vi "Event Logger.vi"(4 "Error IN":errorcluster, 7 "Main VI Base Path IN":path) -> (0 "Error OUT":errorcluster)   [LabVIEW 2018]
uses:
  <vilib>/Utility/file.llb/Write Delimited Spreadsheet (string).vi
  Globals/Global - Configuration Options.vi
panel:
  in  "Headers":string[](array[string])=["Date_Time", "Log Type", "Message"]
  out "Event Log Path":path
  # "INPUTS"
  # "OUTPUTS"
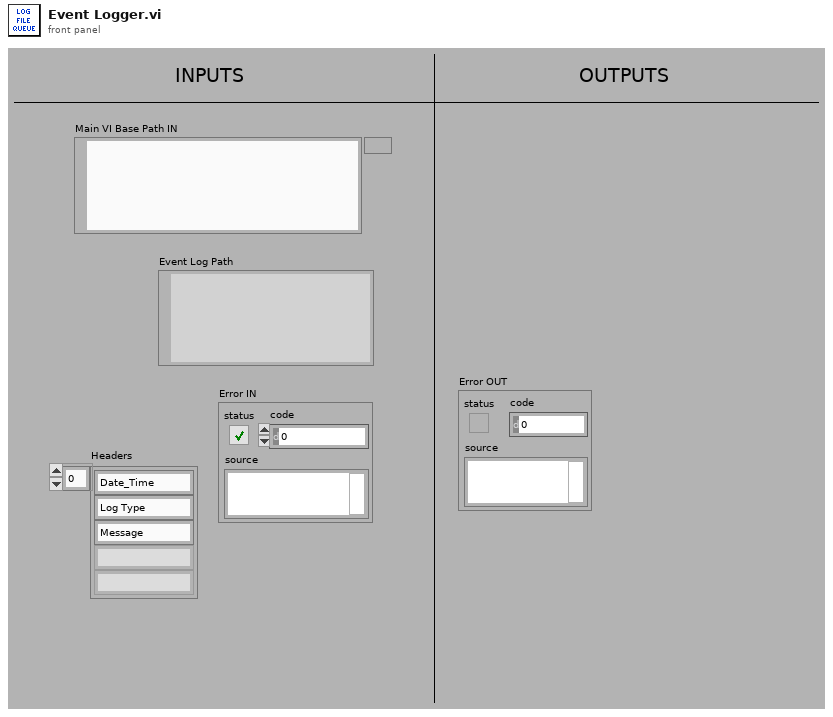
[diagram p1: front panel]
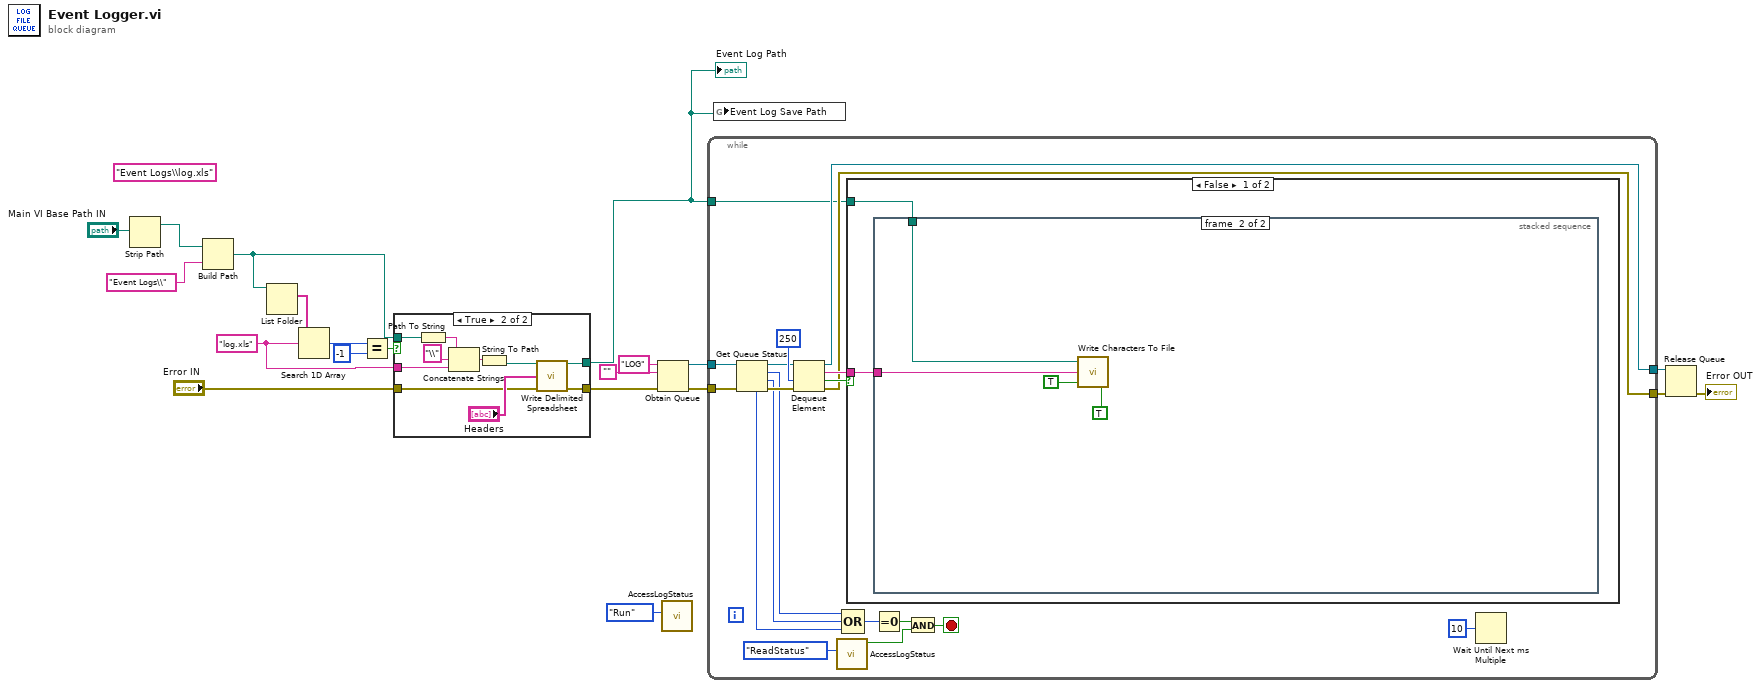
[diagram p0: block diagram]
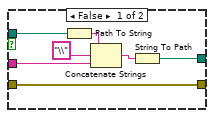
[diagram p2: hidden frame]
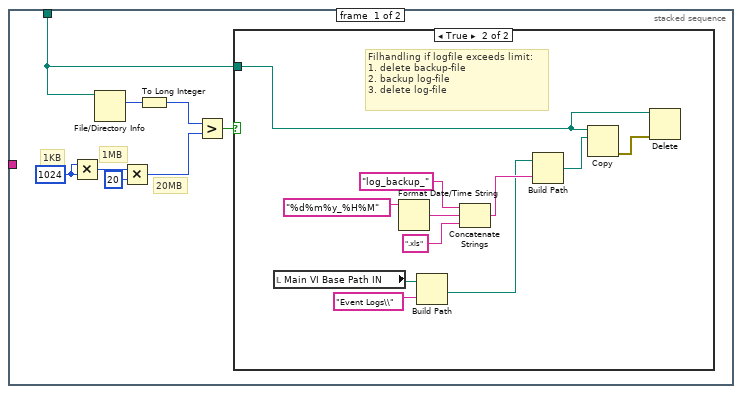
[diagram p3: hidden frame]
diagram:
  (unwired) "Event Logs\\log.xls" ("name or relative path")
  w8 = "log.xls" ("name or relative path")
  n1 = Strip Path(path="Main VI Base Path IN") -> (stripped path=w1:path)  [unwired: 1 out]
  n2 = Build Path(base path=w1, name or relative path="Event Logs\\") -> (appended path=w7:path)
  n3 = List Folder(path=w7) -> (filenames=w4:string[])  [unwired: 1 in, 5 out]
  n4 = Search 1D Array(1D array=w4, element=w8) -> (index of element=w11:i32)  [unwired: 1 out]
  n5 = Equal?(x=w11, y=-1) -> (x = y?=w9:bool)
  n6 = case shown="True" w9 {
    tunnel: w8 -> [w23 w37]
    tunnel: "Error IN" -> [w27 w28]
    tunnel: [w27 w31] -> w6
    tunnel: w7 -> [w21 w35]
    tunnel: [w22 w30] -> w3
    frame False {
      n7 = Path To String(path=w21) -> (string=w25:string)
      n8 = Concatenate Strings(w25, "\\", w23) -> (w26:string)
      n9 = String To Path(string=w26) -> (path=w22:path)
    }
    frame True {
      n10 = Path To String(path=w35) -> (string=w34:string)
      n11 = Concatenate Strings(w34, "\\", w37) -> (w36:string)
      n12 = String To Path(string=w36) -> (path=w29:path)
      n13 = call-poly <vilib>:"Write Delimited Spreadsheet.vi"("file path (dialog if empty)"=w29, "1D data"="Headers", "error in (no error)"=w28) -> ("new file path (Not A Path if cancelled)"=w30:path, "error out"=w31:errorcluster)  [unwired: 11 in]
    }
  }
  "Event Log Path" <- w3
  n14 = Obtain Queue(name (unnamed)="LOG", element data type="", error in (no error)=w6) -> (queue out=w18:refnum<queue>, error out=w17:errorcluster)  [unwired: 2 in, 1 out]
  n15 = call "AccessLogStatus.vi"("Operation"=enum8{"Run", "Stop", "ReadStatus"}."Run") -> ()  [unwired: 6 in, 1 out]
  n16 = while {
    tunnel: w18 -> [w49]
    tunnel: w17 -> [w48]
    tunnel: [w52] -> w16
    tunnel: [w51] -> w15
    tunnel: w3 -> [w38]
    stop <- w39 stop-if-true
    n17 = Get Queue Status(queue=w49, error in (no error)=w48) -> (queue out=w46:refnum<queue>, # pending remove=w43:i32, # pending insert=w44:i32, error out=w47:errorcluster, # elements in queue=w45:i32)  [unwired: 1 in, 3 out]
    n18 = Dequeue Element(queue=w46, timeout in ms (-1)=250, error in (no error)=w47) -> (queue out=w52:refnum<queue>, element=w53:string, timed out?=w54:bool, error out=w51:errorcluster)
    n19 = call "AccessLogStatus.vi"("Operation"=enum8{"Run", "Stop", "ReadStatus"}."ReadStatus") -> ("Status"=w40:bool)  [unwired: 6 in]
    n20 = Compound Arithmetic op=OR(w43, w44, w45) -> (w42:i32)
    n21 = case shown="False" w54 {
      tunnel: w53 -> [w58 _]
      tunnel: w38 -> [w57 _]
      frame False {
        n22 = stacked-sequence {
          tunnel: w57 -> [w60 w78]
          tunnel: w58 -> [_ w80]
          frame #0 {
            w65 = 1024
            # "20MB"
            # "1MB"
            # "1KB"
            n23 = Multiply(x=w65, y=w65) -> (x*y=w64:i32)
            n24 = File/Directory Info(path=w60) -> (size=w59:i64)  [unwired: 1 in, 6 out]
            n25 = Multiply(x=w64, y=20) -> (x*y=w62:i32)
            n26 = To Long Integer(number=w59) -> (32bit integer=w66:i32)
            n27 = Greater?(x=w66, y=w62) -> (0:w61:bool)
            n28 = case shown="True" w61 {
              tunnel: w60 -> [_ w70]
              frame False {
              }
              frame True {
                # "Filhandling if logfile exceeds limit:\n1. delete backup-file\n2. backup log-file\n3. delete log-file"
                n29 = local read "Main VI Base Path IN"() -> (w67:path)
                n30 = Format Date/Time String(time format string (%c)="%d%m%y_%H%M") -> (date/time string=w74:string)  [unwired: 2 in]
                n31 = Build Path(base path=w67, name or relative path="Event Logs\\") -> (appended path=w68:path)
                n32 = Concatenate Strings("log_backup_" ("string"), w74, ".xls" ("string")) -> (w77:string)
                n33 = Build Path(base path=w68, name or relative path=w77) -> (appended path=w72:path)
                n34 = Copy(10:w72, 11:w70) -> (0:w71:errorcluster)  [unwired: 3 in, 2 out]
                n35 = Delete(path (use dialog)=w70, error in=w71) -> ()  [unwired: 3 in, 3 out]
              }
            }
          }
          frame #1 {
            n36 = call <vilib>:"Write Characters To File.vi"("convert eol? (no:F)"=TRUE, "append to file? (new file:F)"=TRUE, "character string"=w80, "file path (dialog if empty)"=w78) -> ()  [unwired: 1 in, 1 out]
          }
        }
      }
      frame True {
      }
    }
    n37 = Equal To 0?(x=w42) -> (x = 0?=w41:bool)
    n38 = And(x=w41, y=w40) -> (x .and. y?=w39:bool)
    n39 = Wait Until Next ms Multiple(millisecond multiple=u32 10) -> ()  [unwired: 1 out]
  }
  n40 = global write "Global - Configuration Options.vi" "Event Log Save Path"(w3) -> ()
  n41 = Release Queue(queue=w16, error in (no error)=w15) -> (error out=→"Error OUT":errorcluster)  [unwired: 1 in, 2 out]
